vi "Get Attribute I32.vi"(8 "error in":errorcluster, 10 "Attribute":string, 11 "Config from XML in":refnum<class "Config from XML.lvclass">) -> (0 "error out":errorcluster, 2 "Value":i32, 3 "Config from XML out":refnum<class "Config from XML.lvclass">)   [LabVIEW 2025, in "Config from XML.lvclass"]
uses:
  Config from XML.lvclass
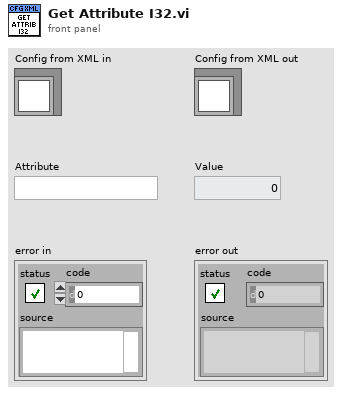
[diagram p1: front panel]
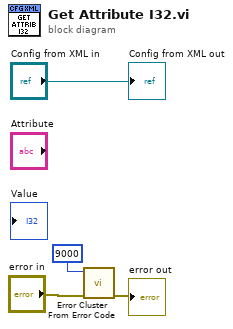
[diagram p0: block diagram]
diagram:
  n1 = call <vilib>:"Error Cluster From Error Code.vi"("error in (no error)"="error in", "error code (0)"=9000) -> ("error out"=→"error out":errorcluster)  [unwired: 7 in]
  "Config from XML out" <- "Config from XML in"
